vi "Test MQTT-2.3.1-2.vi"(8 "error in (no error)":errorcluster) -> (0 "error out":errorcluster)   [LabVIEW 2013]
uses:
  source/Control Packets/SUBSCRIBE/Topic Subscription -- cluster.ctl
  source/Control Packets/ControlPacket/QualityOfService -- enum.ctl
  source/Control Packets/ControlPacket/ControlPacket.lvclass/ControlPacket.ctl
  <vilib>/addons/_JKI Toolkits/Caraya/classes/Test/Test.lvclass
  <vilib>/addons/_JKI Toolkits/Caraya/classes/Assert/Assert.lvclass
  source/Control Packets/PUBLISH/PUBLISH.lvclass
  source/Control Packets/SUBSCRIBE/SUBSCRIBE.lvclass
  source/Control Packets/UNSUBSCRIBE/UNSUBSCRIBE.lvclass
  source/Control Packets/ControlPacket/ControlPacket.lvclass
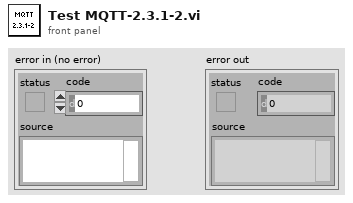
[diagram p1: front panel]
types:
  T1 = typedef "SUBSCRIBE.lvclass/Topic Subscription -- cluster.ctl" = cluster{"Topic Filter":string, "QoS":T2}
  T2 = typedef "ControlPacket.lvclass/QualityOfService -- enum.ctl" = enum16{"0 (At Most Once)", "1 (At Least Once)", "2 (Exactly Once)"}
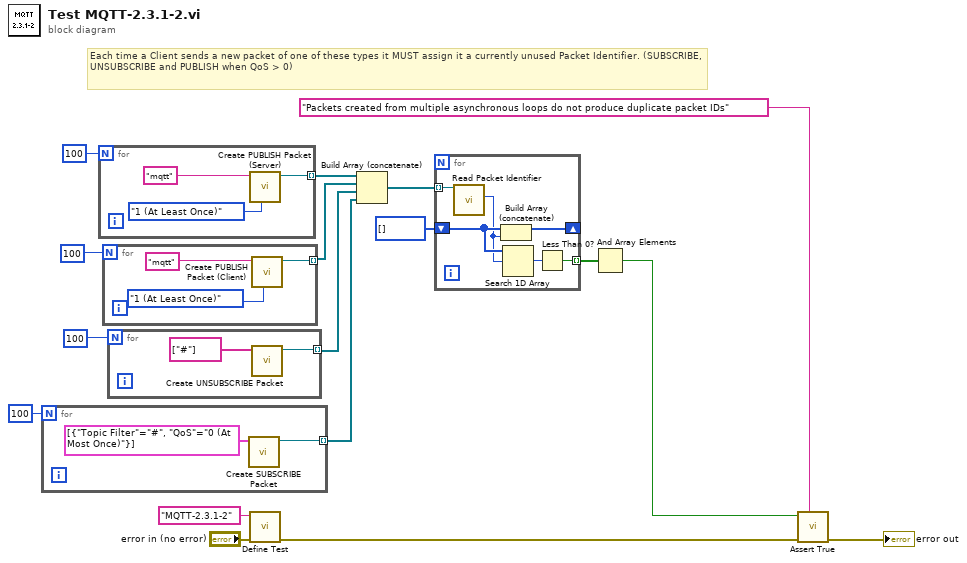
[diagram p0: block diagram]
diagram:
  # "Each time a Client sends a new packet of one of these types it MUST assign it a currently unused Packet Identifier. (SUBSCRIBE, UNSUBSCRIBE and PUBLISH when QoS > 0)"
  n1 = for {
    N: 100 -> [_]
    tunnel: [w19] -> w5 mode=indexing
    n2 = call "Create SUBSCRIBE Packet.vi"("Topic Subscriptions"=T1[] [{"Topic Filter"="#", "QoS"=enum."0 (At Most Once)"}]) -> ("SUBSCRIBE out"=w19:refnum<class "SUBSCRIBE.lvclass">)  [unwired: 9 in, 1 out]
  }
  n3 = for {
    N: 100 -> [_]
    tunnel: [w20] -> w8 mode=indexing
    n4 = call "Create PUBLISH Packet (Server).vi"("QoS"=QualityOfService_--_enum."1 (At Least Once)", "Topic Name"="mqtt") -> ("PUBLISH"=w20:refnum<class "PUBLISH.lvclass">)  [unwired: 7 in, 2 out]
  }
  n5 = for {
    N: 100 -> [_]
    tunnel: [w23] -> w7 mode=indexing
    n6 = call "Create PUBLISH Packet (Client).vi"("QoS"=QualityOfService_--_enum."1 (At Least Once)", "Topic Name"="mqtt") -> ("PUBLISH"=w23:refnum<class "PUBLISH.lvclass">)  [unwired: 7 in, 2 out]
  }
  n7 = for {
    N: 100 -> [_]
    tunnel: [w26] -> w6 mode=indexing
    n8 = call "Create UNSUBSCRIBE Packet.vi"("Topic Subscriptions"=string[] ["#"]) -> ("UNSUBSCRIBE out"=w26:refnum<class "UNSUBSCRIBE.lvclass">)  [unwired: 9 in, 1 out]
  }
  n9 = call <vilib>:"Define Test.vi"("error in (no error)"="error in (no error)", "Label (VI Title)"="MQTT-2.3.1-2") -> ("error out"=w15:errorcluster)  [unwired: 9 in]
  n10 = Build Array (concatenate)(w8, w7, w6, w5) -> (w4:refnum<class "ControlPacket.lvclass">[])
  n11 = for {
    tunnel: w4 -> [w33] mode=indexing
    shift-right: [w32] -> _
    shift-left: u16[] [] -> [w31]
    tunnel: [w28] -> w2 mode=indexing
    n12 = call "Read Packet Identifier.vi"("ControlPacket in"=w33) -> ("Packet Identifier"=w30:u16)  [unwired: 9 in, 1 out]
    n13 = Build Array (concatenate)(w31, w30) -> (w32:u16[])
    n14 = Search 1D Array(1D array=w31, element=w30) -> (index of element=w29:i32)  [unwired: 1 in]
    n15 = Less Than 0?(x=w29) -> (x < 0?=w28:bool)
  }
  n16 = And Array Elements(Boolean array=w2) -> (logical AND=w1:bool)
  n17 = call <vilib>:"Assert True.vi"("Label"="Packets created from multiple asynchronous loops do not produce duplicate packet IDs", "error in (no error)"=w15, "True?"=w1) -> ("error out"=→"error out":errorcluster)  [unwired: 8 in]
